vi "SetFontColor.vi"(5 "列":i32, 7 "行":i32, 8 "error":errorcluster caption="错误输入（无错误）", 9 "取消字体颜色":bool, 10 "颜色盒":u32(colorbox), 11 "Excel._Worksheet":refnum<k7>) -> (0 "error out":errorcluster caption="错误输出", 3 "Excel._Worksheet":refnum<k7>)   [LabVIEW 2014]
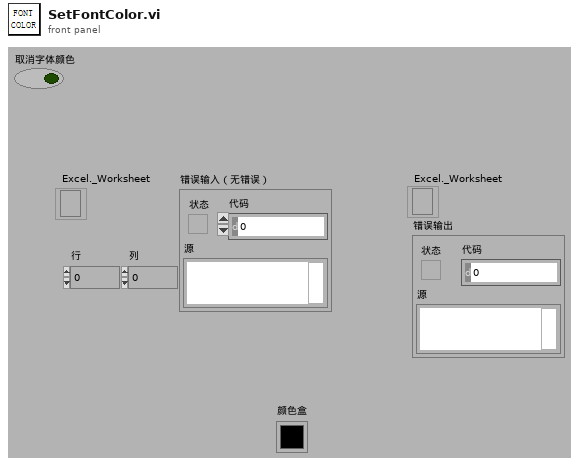
[diagram p1: front panel]
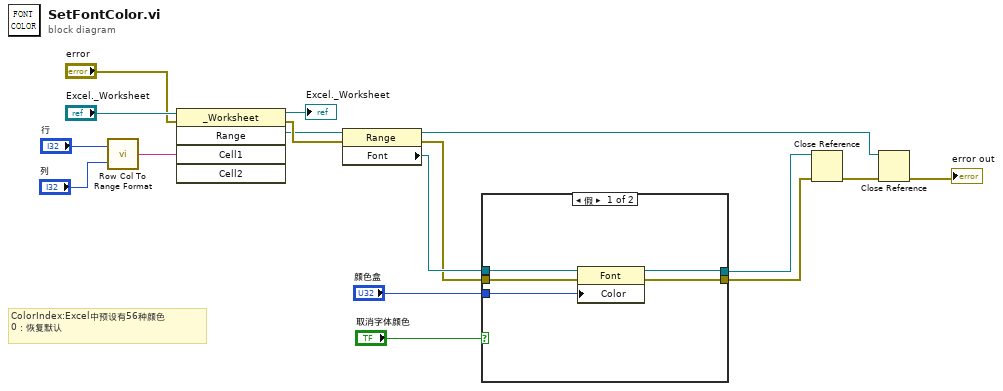
[diagram p0: block diagram]
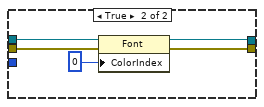
[diagram p2: hidden frame]
diagram:
  # "ColorIndex:Excel中预设有56种颜色\n0：恢复默认"
  n1 = call "Row Col To Range Format.vi"("Column"="列", "Row"="行") -> ("Output String"=w1:string)
  n2 = invoke class="_Worksheet" method="Range"(reference="Excel._Worksheet", error in="error", "Cell1"=w1) -> (reference out=→"Excel._Worksheet":refnum<k7>, error out=w13:errorcluster, "Range"=w11:refnum<k7>)  [unwired: 2 in, 2 out]
  n3 = property class="Range"(reference=w11, error in=w13) -> (reference out=w9:refnum<k7>, error out=w4:errorcluster, "Font"=w5:refnum<k7>)
  n4 = case shown="假" "取消字体颜色" {
    tunnel: [w21 w27] -> w7
    tunnel: w5 -> [w22 w26]
    tunnel: w4 -> [w20 w25]
    tunnel: [w19 w24] -> w3
    tunnel: "颜色盒" -> [w18 _]
    frame False {
      n5 = property class="Font"(reference=w22, error in=w20, "Color"=w18) -> (reference out=w21:refnum<k7>, error out=w19:errorcluster)
    }
    frame True {
      n6 = property class="Font"(reference=w26, error in=w25, "ColorIndex"=0) -> (reference out=w27:refnum<k7>, error out=w24:errorcluster)
    }
  }
  n7 = Close Reference(reference=w7, error in (no error)=w3) -> (error out=w10:errorcluster)
  n8 = Close Reference(reference=w9, error in (no error)=w10) -> (error out=→"error out":errorcluster)
